vi "Hashes Example.vi"() -> (0 "error out":errorcluster, 1 "set = get?":bool, 2 "# of fields added":i64, 5 "KEY":string)   [LabVIEW 2019, in "Redis Client Examples.lvlib"]
uses:
  Redis Client Examples.lvlib
  <vilib>/numeric/Random Number (Range) I64.vi
  <vilib>/numeric/sub_Random U32.vi
  Redis Client for LabVIEW/Redis Pipelining TCP Client/Redis Pipelining TCP Client.lvclass
  C:/Users/Nicholas Folse/Documents/workspace/github-tauterra.llc/Redis Client for LabVIEW/Redis Client for LabVIEW/Redis Client/Redis Client.lvclass
  Redis Client for LabVIEW/Redis Pipelining TCP Client/impl/set pipelining.vi
  lib/RESP3-for-LabVIEW/RESP3/high-level/RESP3 Get String.vi
  Redis Client for LabVIEW/Redis Client/Redis Client.lvclass
  Redis Client for LabVIEW/Redis TCP Client/Redis TCP Client.lvclass
  lib/RESP3-for-LabVIEW/RESP3/RESP3.lvlib
  C:/Users/Nicholas Folse/Documents/workspace/github-tauterra.llc/Redis Client for LabVIEW/Redis Client for LabVIEW/Redis TCP Client/Redis TCP Client.lvclass
panel:
  out "ping response":variant
  out "server properties":variant
  out "client name":string
  out "client info":string
  out "client id":i64 format="%.0x"
  out "Pipeline: RESP3 Values":variant[](array[variant])
  in  "pipelining enabled?":bool=TRUE
  out "execution time (ms/key)":dbl
  in  "# of keys to test":i32=500
  out "all keys found?":bool
  out "iter#":i32=49
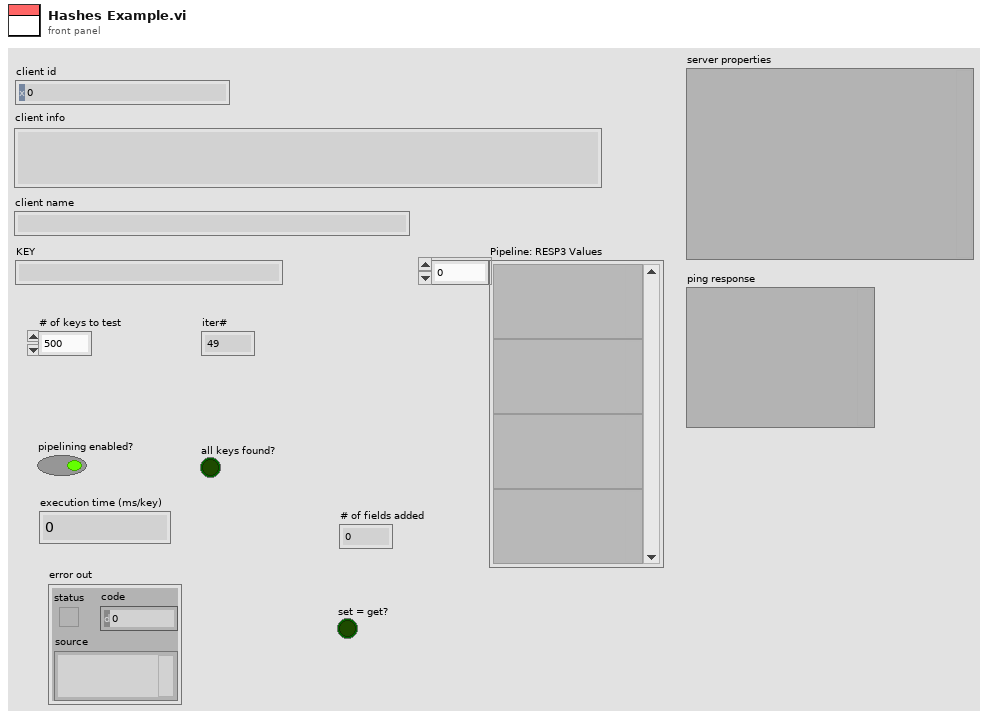
[diagram p1: front panel]
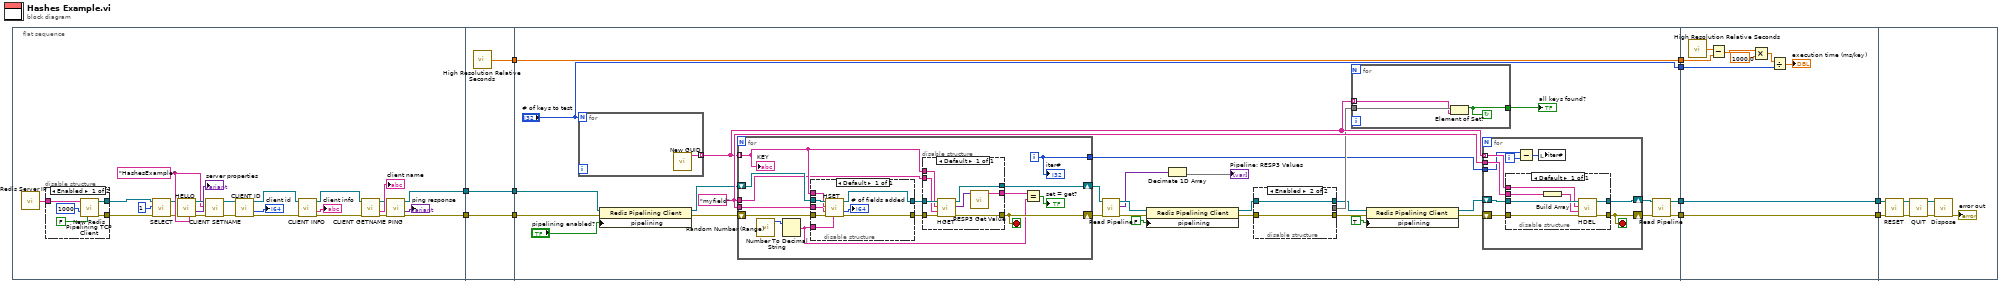
[diagram p0: block diagram]
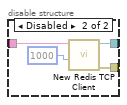
[diagram p2: hidden frame]
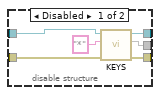
[diagram p3: hidden frame]
diagram:
  n1 = flat-sequence {
    tunnel: [w19] -> w7
    tunnel: [w20] -> w5
    tunnel: [w47] -> w10
    tunnel: [w46] -> w8
    tunnel: w7 -> [w46]
    tunnel: [w45] -> w6
    tunnel: w5 -> [w45]
    tunnel: [w72] -> w11
    tunnel: w10 -> [w72]
    tunnel: ["# of keys to test"] -> w9
    tunnel: w8 -> [w51]
    tunnel: w6 -> [w50]
    tunnel: [w49] -> w3
    tunnel: [w48] -> w1
    tunnel: w11 -> [w143]
    tunnel: w9 -> [w138]
    tunnel: [w137] -> w4
    tunnel: w3 -> [w137]
    tunnel: [w136] -> w2
    tunnel: w1 -> [w136]
    tunnel: w4 -> [w148]
    tunnel: w2 -> [w149]
    frame #0 {
      w23 = "HashesExample" ("client name")
      n2 = call "Redis Server IP.vi"() -> ("server IP"=w24:string)
      n3 = disable-structure shown="Enabled" {
        disable-tunnel: w24 -> [w40 w44]
        disable-tunnel: [w39 w42] -> w15
        disable-tunnel: [w38 w41] -> w16
        frame Enabled {
          n4 = call "New Redis Pipelining TCP Client.vi"("pipelining enabled?"=FALSE, "timeout ms (25000)"=1000, "address"=w40) -> ("error out"=w39:errorcluster, "Redis Pipelining TCP Client out"=w38:refnum<class "Redis Pipelining TCP Client.lvclass">)  [unwired: 7 in]
        }
        frame Disabled {
          n5 = call "New Redis TCP Client.vi"("timeout ms (25000)"=1000, "address"=w44) -> ("error out"=w42:errorcluster, "Redis TCP Client out"=w41:refnum<class "Redis TCP Client.lvclass">)  [unwired: 8 in]
        }
      }
      n6 = call "SELECT.vi"("error in (no error)"=w15, "index"=i64 1, "Redis Client in"=w16) -> ("error out"=w13:errorcluster, "Redis Client out"=w14:refnum<class "Redis Pipelining TCP Client.lvclass">)  [unwired: 6 in, 1 out]
      n7 = call "HELLO.vi"("client name"=w23, "error in (no error)"=w13, "Redis Client in"=w14) -> ("error out"=w33:errorcluster, "server properties"=→"server properties":variant, "Redis Client out"=w34:refnum<class "Redis Pipelining TCP Client.lvclass">)  [unwired: 6 in]
      n8 = call "CLIENT SETNAME.vi"("error in (no error)"=w33, "client name"=w23, "Redis Client in"=w34) -> ("error out"=w32:errorcluster, "Redis Client out"=w31:refnum<class "Redis Pipelining TCP Client.lvclass">)  [unwired: 6 in, 1 out]
      n9 = call "CLIENT ID.vi"("error in (no error)"=w32, "Redis Client in"=w31) -> ("error out"=w27:errorcluster, "client id"=→"client id":i64, "Redis Client out"=w26:refnum<class "Redis Pipelining TCP Client.lvclass">)  [unwired: 7 in]
      n10 = call "CLIENT INFO.vi"("error in (no error)"=w27, "Redis Client in"=w26) -> ("error out"=w30:errorcluster, "client info"=→"client info":string, "Redis Client out"=w29:refnum<class "Redis Pipelining TCP Client.lvclass">)  [unwired: 7 in]
      n11 = call "CLIENT GETNAME.vi"("error in (no error)"=w30, "Redis Client in"=w29) -> ("error out"=w18:errorcluster, "client name"=→"client name":string, "Redis Client out"=w21:refnum<class "Redis Pipelining TCP Client.lvclass">)  [unwired: 7 in]
      n12 = call "PING.vi"("error in (no error)"=w18, "Redis Client in"=w21) -> ("error out"=w19:errorcluster, "response"=→"ping response":variant, "Redis Client out"=w20:refnum<class "Redis Pipelining TCP Client.lvclass">)  [unwired: 7 in]
    }
    frame #1 {
      n13 = call <vilib>:"High Resolution Relative Seconds.vi"() -> ("relative seconds"=w47:dbl)
    }
    frame #2 {
      w77 = "myfield" ("field")
      n14 = for {
        N: "# of keys to test" -> [_]
        tunnel: [w102] -> w76 mode=indexing
        n15 = call "New GUID.vi"() -> ("ToString"=w102:string)  [unwired: 11 in]
      }
      n16 = property class="Redis Pipelining Client"(reference=w50, error in=w51, "pipelining"="pipelining enabled?") -> (reference out=w54:refnum<class "Redis Pipelining TCP Client.lvclass">, error out=w52:errorcluster)
      n17 = for {
        shift-right: [w109] -> w70
        shift-left: w54 -> [w116]
        shift-right: [w105] -> w69
        shift-left: w52 -> [w115]
        tunnel: w76 -> [w110] mode=indexing
        tunnel: w77 -> [w108]
        tunnel: w77 -> [w107]
        tunnel: [w106] -> w73
        i -> [w106]
        stop <- w105 stop-if-true
        n18 = call-poly <vilib>:"Random Number (Range).vi"() -> ("number"=w104:i64)  [unwired: 11 in]
        n19 = Number To Decimal String(number=w104) -> (decimal integer string=w103:string)  [unwired: 1 in]
        n20 = disable-structure shown="Default" {
          disable-tunnel: w116 -> [w132]
          disable-tunnel: w115 -> [w131]
          disable-tunnel: [w130] -> w114
          disable-tunnel: [w129] -> w113
          disable-tunnel: w110 -> [w127]
          disable-tunnel: w107 -> [w126]
          disable-tunnel: w103 -> [w125]
          frame Enabled {
            n21 = call "HSET.vi"("string value"=w125, "error in (no error)"=w131, "field"=w126, "key"=w127, "Redis Client in"=w132) -> ("error out"=w129:errorcluster, "# of fields added"=→"# of fields added":i64, "Redis Client out"=w130:refnum<class "Redis Pipelining TCP Client.lvclass">)  [unwired: 4 in]
          }
        }
        n22 = disable-structure shown="Default" {
          disable-tunnel: w114 -> [w124]
          disable-tunnel: [w123] -> w105
          disable-tunnel: [w122] -> w109
          disable-tunnel: w113 -> [w121]
          disable-tunnel: [w118] -> w112
          disable-tunnel: w110 -> [w120]
          disable-tunnel: w108 -> [w119]
          frame Enabled {
            n23 = call "HGET.vi"("error in (no error)"=w121, "field"=w119, "key"=w120, "Redis Client in"=w124) -> ("error out"=w123:errorcluster, "RESP3 Value"=w117:variant, "Redis Client out"=w122:refnum<class "Redis Pipelining TCP Client.lvclass">)  [unwired: 4 in, 1 out]
            n24 = call-poly "RESP3 Get Value.vi"("RESP3 Value in"=w117) -> ("String out"=w118:string)  [unwired: 7 in, 3 out]
          }
        }
        n25 = Equal?(x=w112, y=w103) -> (x = y?=→"set = get?":bool)
        "KEY" <- w110
        "iter#" <- w106
      }
      n26 = call "Read Pipeline.vi"("error in (no error)"=w69, "Redis Pipelining Client in"=w70) -> ("error out"=w61:errorcluster, "RESP3 Values"=w56:variant[], "Redis Pipelining Client out"=w68:refnum<class "Redis Pipelining TCP Client.lvclass">)  [unwired: 6 in, 1 out]
      n27 = property class="Redis Pipelining Client"(reference=w68, error in=w61, "pipelining"=FALSE) -> (reference out=w64:refnum<class "Redis Pipelining TCP Client.lvclass">, error out=w60:errorcluster)
      n28 = Decimate 1D Array(w56) -> (→"Pipeline: RESP3 Values":variant[])  [unwired: 1 out]
      n29 = disable-structure shown="Enabled" {
        disable-tunnel: [w82 _] -> w75
        disable-tunnel: [w81 w85] -> w65
        disable-tunnel: w64 -> [w80 w85]
        disable-tunnel: [w79 w84] -> w62
        disable-tunnel: w60 -> [w78 w84]
        frame Disabled {
          n30 = call "KEYS.vi"("error in (no error)"=w78, "pattern"="*", "Redis Client in"=w80) -> ("error out"=w79:errorcluster, "keys"=w82:set{string}, "Redis Client out"=w81:refnum<class "Redis Pipelining TCP Client.lvclass">)  [unwired: 6 in]
        }
        frame Enabled {
        }
      }
      n31 = for {
        tunnel: w76 -> [w134] mode=indexing
        tunnel: w75 -> [w135]
        tunnel: [w133] -> w74
        stop <- w133 continue-if-true
        n32 = Element of Set?(10:w134, 11:w135) -> (3:w133:bool)
      }
      "all keys found?" <- w74
      n33 = property class="Redis Pipelining Client"(reference=w65, error in=w62, "pipelining"=TRUE) -> (reference out=w63:refnum<class "Redis Pipelining TCP Client.lvclass">, error out=w59:errorcluster)
      n34 = for {
        shift-right: [w94] -> w67
        shift-left: w63 -> [w90]
        shift-right: [w86] -> w66
        shift-left: w59 -> [w93]
        tunnel: w76 -> [w92] mode=indexing
        tunnel: w77 -> [w91]
        tunnel: w73 -> [w88]
        i -> [w89]
        stop <- w86 stop-if-true
        n35 = disable-structure shown="Default" {
          disable-tunnel: w90 -> [w101]
          disable-tunnel: w93 -> [w100]
          disable-tunnel: [w99] -> w94
          disable-tunnel: [w98] -> w86
          disable-tunnel: w92 -> [w97]
          disable-tunnel: w91 -> [w96]
          frame Enabled {
            n36 = Build Array(w96) -> (w95:string[])
            n37 = call "HDEL.vi"("error in (no error)"=w100, "fields"=w95, "key"=w97, "Redis Client in"=w101) -> ("error out"=w98:errorcluster, "Redis Client out"=w99:refnum<class "Redis Pipelining TCP Client.lvclass">)  [unwired: 5 in, 1 out]
          }
        }
        n38 = Subtract(x=w88, y=w89) -> (x-y=w87:i32)
        n39 = local write "iter#"(w87) -> ()
      }
      n40 = call "Read Pipeline.vi"("error in (no error)"=w66, "Redis Pipelining Client in"=w67) -> ("error out"=w49:errorcluster, "Redis Pipelining Client out"=w48:refnum<class "Redis Pipelining TCP Client.lvclass">)  [unwired: 6 in, 2 out]
    }
    frame #3 {
      n41 = call <vilib>:"High Resolution Relative Seconds.vi"() -> ("relative seconds"=w144:dbl)
      n42 = Subtract(x=w144, y=w143) -> (x-y=w142:dbl)
      n43 = Multiply(x=w142, y=1000.0) -> (x*y=w140:dbl)
      n44 = Divide(x=w140, y=w138) -> (x/y=→"execution time (ms/key)":dbl)
    }
    frame #4 {
      n45 = call "RESET.vi"("error in (no error)"=w148, "Redis Client in"=w149) -> ("error out"=w147:errorcluster, "Redis Client out"=w150:refnum<class "Redis Pipelining TCP Client.lvclass">)  [unwired: 8 in]
      n46 = call "QUIT.vi"("error in (no error)"=w147, "Redis Client in"=w150) -> ("error out"=w146:errorcluster, "Redis Client out"=w145:refnum<class "Redis Pipelining TCP Client.lvclass">)  [unwired: 8 in]
      n47 = call-dynamic "Dispose.vi"("error in (no error)"=w146, "Redis Pipelining TCP Client in"=w145) -> ("error out"=→"error out":errorcluster)  [unwired: 9 in]
    }
  }
